vi "32bit-to-16bit.vi"(1 "32位寄存器值":i32[](array[numeric]) format="%x") -> (0 "16位寄存器值":u16[](array[numeric]) format="%x")   [LabVIEW 2023]
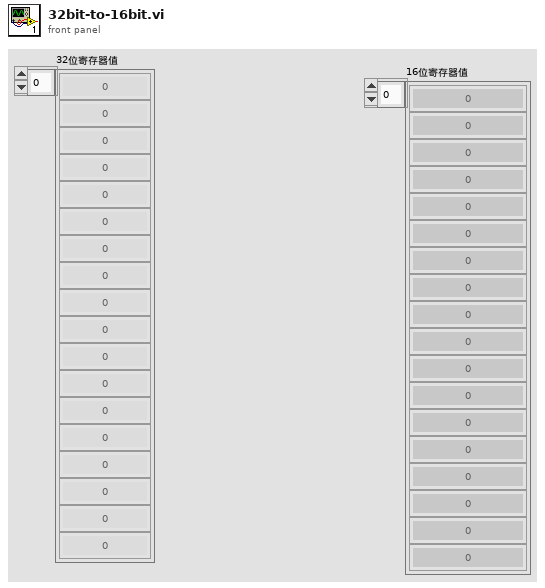
[diagram p1: front panel]
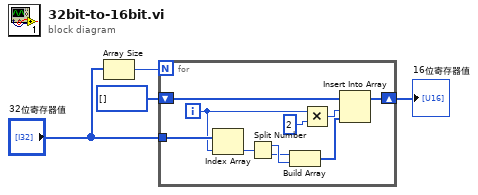
[diagram p0: block diagram]
diagram:
  n1 = Array Size(array="32位寄存器值") -> (size(s)=w1:i32)
  n2 = for {
    N: w1 -> [_]
    tunnel: "32位寄存器值" -> [w14]
    shift-right: [w6] -> w4
    shift-left: i32[] [] -> [w5]
    i -> [w9]
    n3 = Index Array(array=w14, index=w9) -> (element=w13:i32)
    n4 = Split Number(x=w13) -> (hi(x)=w12:u16, lo(x)=w11:u16)
    n5 = Build Array(w11, w12) -> (w10:u16[])
    n6 = Multiply(x=w9, y=2) -> (x*y=w7:i32)
    n7 = Insert Into Array(array=w5, index=w7, new element=w10) -> (w6:i32[])
  }
  "16位寄存器值" <- w4
